vi "getDtFromXml.vi"(8 "error in (no error)":errorcluster, 10 "Xml":refnum<class "xmlNode.lvclass">, 11 "ScriptEvent in":refnum<class "ScriptEvent.lvclass">) -> (0 "error out":errorcluster, 2 "Xml out":refnum<class "xmlNode.lvclass">, 3 "ScriptEvent out":refnum<class "ScriptEvent.lvclass">)   [LabVIEW 2009, in "Tools.lvlib" / "Scripting.lvlib" / "ScriptEvent.lvclass"]
uses:
  ScriptEvent.lvclass
  xmlNode/xmlNode.lvclass
  ScriptEvent.lvclass/ScriptEvent.ctl
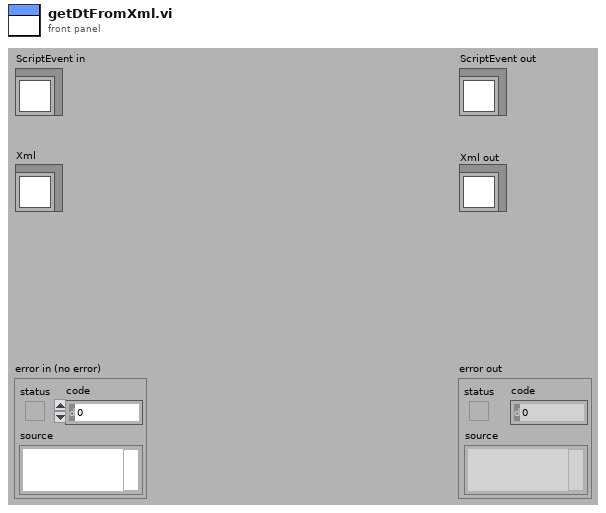
[diagram p1: front panel]
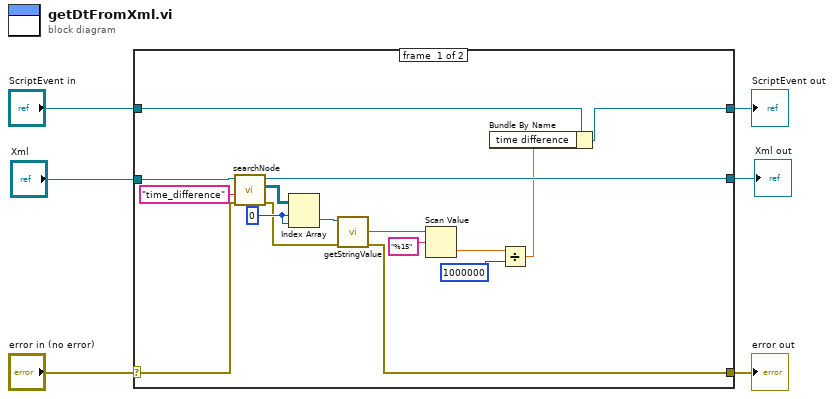
[diagram p0: block diagram]
diagram:
  n1 = case shown="No Error" "error in (no error)" {
    selector: "error in (no error)" -> [w11 w24]
    tunnel: [w12 w24] -> w5
    tunnel: [w14 w23] -> w3
    tunnel: "ScriptEvent in" -> [w15 w23]
    tunnel: "Xml" -> [w22 _]
    tunnel: [w13 _] -> w1
    frame #0 {
      w19 = 0
      n2 = call-dynamic "searchNode.vi"("error in (no error)"=w11, "searchElementName"="time_difference", "xmlNode in"=w22) -> ("error out"=w10:errorcluster, "arrayXmlNodes"=w20:refnum<class "xmlNode.lvclass">[][], "xmlNode out"=w13:refnum<class "xmlNode.lvclass">)  [unwired: 6 in]
      n3 = Index Array(array=w20, index (row)=w19, index (col)=w19) -> (element=w18:refnum<class "xmlNode.lvclass">)
      n4 = call-dynamic "getStringValue.vi"("error in (no error)"=w10, "xmlNode.lvclass in"=w18) -> ("error out"=w12:errorcluster, "stringValue"=w17:string)  [unwired: 7 in, 1 out]
      n5 = Scan Value(string=w17, format string="%15") -> (value=w8:dbl)  [unwired: 1 in, 1 out]
      n6 = Divide(x=w8, y=1000000) -> (x/y=w7:dbl)
      n7 = Bundle By Name(cluster=w15, "time difference"=w7) -> (w14:refnum<class "ScriptEvent.lvclass">)
    }
    frame #1 {
    }
  }
  "error out" <- w5
  "ScriptEvent out" <- w3
  "Xml out" <- w1
